vi "Request voltage CH1 (SubVI).vi"() -> (3 "Request voltage CH1 / X":string)   [LabVIEW 2018]
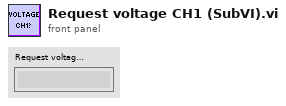
[diagram p1: front panel]
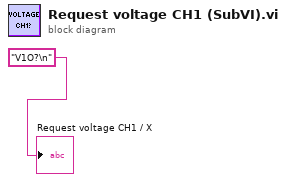
[diagram p0: block diagram]
diagram:
  "Request voltage CH1 / X" <- "V1O?\n" ("format string")
